vi "Get Speed.vi"(8 "error in (no error)":errorcluster, 10 "Axis Name":string, 11 "iMotion Controller in":refnum<class "iMotion Controller.lvclass">) -> (0 "error out":errorcluster, 2 "Axis Speed":dbl, 3 "iMotion Controller out":refnum<class "iMotion Controller.lvclass">)   [LabVIEW 2022 SP3, in "iMotion Controller.lvclass"]
uses:
  iMotion Controller.lvclass
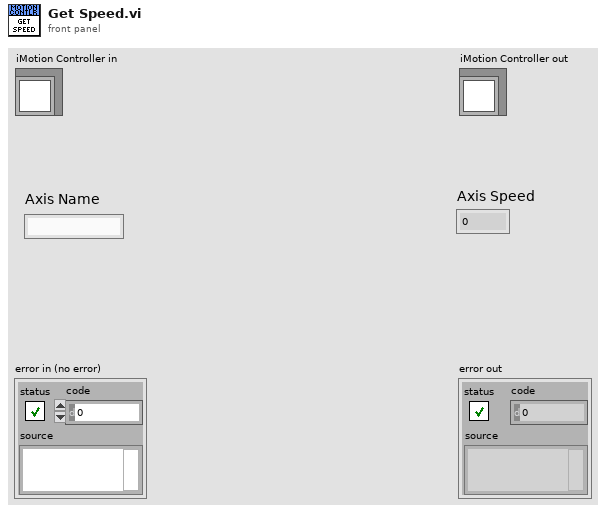
[diagram p1: front panel]
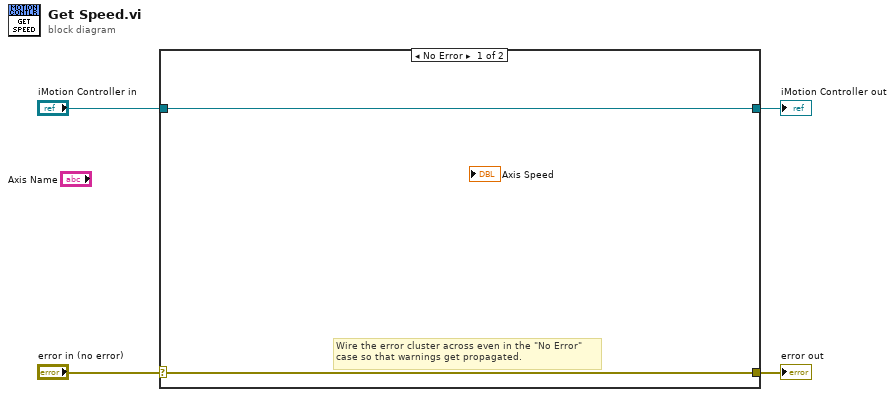
[diagram p0: block diagram]
diagram:
  n1 = case shown="No Error" "error in (no error)" {
    selector: "error in (no error)" -> [w5 w8]
    tunnel: [w5 w8] -> w3
    tunnel: [w6 w7] -> w1
    tunnel: "iMotion Controller in" -> [w6 w7]
    frame No Error {
      # "Wire the error cluster across even in the \"No Error\"\ncase so that warnings get propagated."
    }
    frame Error {
    }
  }
  "error out" <- w3
  "iMotion Controller out" <- w1
